vi "Main.vi"() -> ()   [LabVIEW 2020, in "LV Server.lvclass"]
uses:
  LV Server.lvclass
  LV Server.lvclass/LV Server.ctl
panel:
  in  "TCP Port":u16=4763
  out "Error":errorcluster
  in  "WS Port":u16=4663
  in  "HTTP Port":u16=7080
  # "Modify the above ports if necessary and then run this VI to start the server."
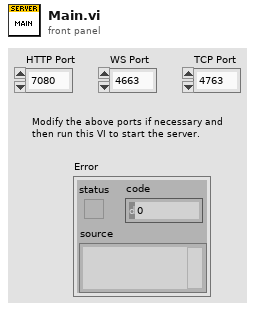
[diagram p1: front panel]
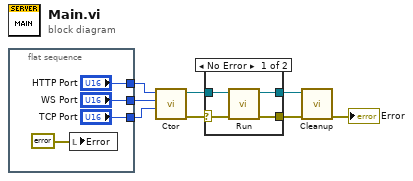
[diagram p0: block diagram]
diagram:
  n1 = flat-sequence {
    tunnel: ["HTTP Port"] -> w4
    tunnel: ["WS Port"] -> w3
    tunnel: ["TCP Port"] -> w1
    frame #0 {
      n2 = local write "Error"(errorcluster {"status"=FALSE, "code"=0, "source"=""} ("error out")) -> ()
    }
  }
  n3 = call "Ctor.vi"("TCP Port"=w1, "WS Port"=w3, "HTTP Port"=w4) -> ("error out"=w8:errorcluster, "LV Server out"=w7:refnum<class "LV Server.lvclass">)  [unwired: 7 in]
  n4 = case shown="No Error" w8 {
    selector: w8 -> [w15 w18]
    tunnel: w7 -> [w16 w17]
    tunnel: [w14 w17] -> w5
    tunnel: [w13 w18] -> w6
    frame No Error {
      n5 = call "Run.vi"("error in (no error)"=w15, "LV Server in"=w16) -> ("error out"=w13:errorcluster, "LV Server out"=w14:refnum<class "LV Server.lvclass">)  [unwired: 8 in]
    }
    frame Error {
    }
  }
  n6 = call "Cleanup.vi"("error in (no error)"=w6, "LV Server in"=w5) -> ("error out"=→"Error":errorcluster)  [unwired: 9 in]
